vi "numCmd_Recv_Array.vi"(7 "Command Name":string, 11 "Initial Values":dbl[](array[numeric])) -> (0 "error out":errorcluster, 2 "Any Changed":bool, 3 "Values":dbl[](array[numeric]))   [LabVIEW 2019, in "Trajectory_Library.lvlib"]
uses:
  Trajectory_Library.lvlib
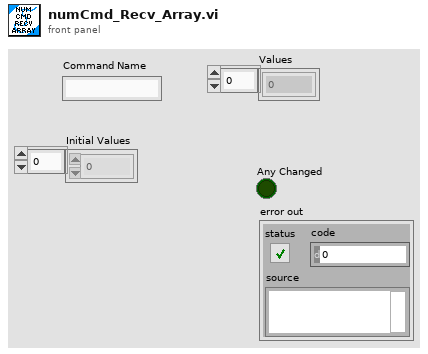
[diagram p1: front panel]
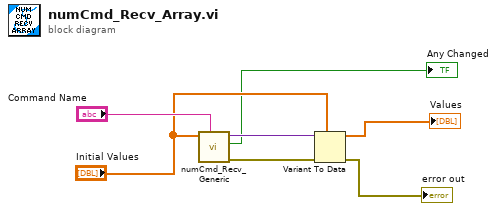
[diagram p0: block diagram]
diagram:
  n1 = call "numCmd_Recv_Generic.vi"("Command Name"="Command Name", "Initial Value"="Initial Values") -> ("error out"=w7:errorcluster, "Changed"=→"Any Changed":bool, "Newest Value"=w2:variant)  [unwired: 7 in]
  n2 = Variant To Data(error in=w7, type="Initial Values", Variant=w2) -> (data=→"Values":dbl[], error out=→"error out":errorcluster)
